vi "Check Generation Status.vi"(0 "fpga interface in":refnum<k20>, 11 "error in (no error)":errorcluster) -> (4 "fpga interface out":refnum<k20>, 6 "generation done":bool, 8 "generation state":T1(ring), 15 "error out":errorcluster)   [LabVIEW 2023, in "GettingStarted_Gen_148X_Host.lvlib"]
uses:
  GettingStarted_Gen_148X_Host.lvlib
  <instrlib>/FlexRIO/CSI-2/v2/FPGA/Types/Generation Engine State.ctl
  <instrlib>/FlexRIO/CSI-2/v2/FPGA/NI CSI-2 API FPGA v2.lvlib
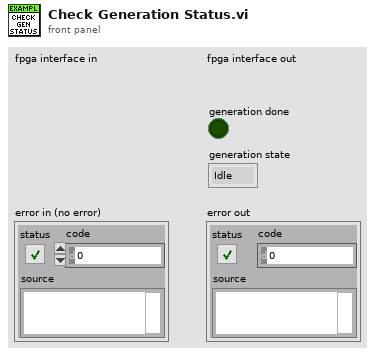
[diagram p1: front panel]
types:
  T1 = enum8{"Idle", "Ready For Start Trigger", "Generate Packets", "Done", "Error"}
  T2 = typedef "NI CSI-2 API FPGA v2.lvlib/Generation Engine State.ctl" = enum8{"Idle", "Ready For Start Trigger", "Generate Packets", "Done", "Error"}
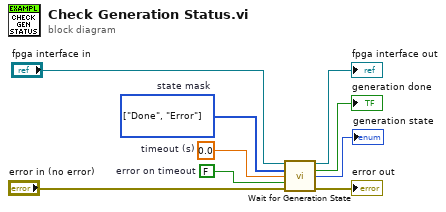
[diagram p0: block diagram]
diagram:
  w4 = FALSE  # error on timeout
  w5 = 0.0  # timeout (s)
  w6 = T2[] [enum."Done", enum."Error"] items=["Idle", "Ready For Start Trigger", "Generate Packets", "Done", "Error"]  # state mask
  n1 = call "Wait for Generation State.vi"("fpga interface in"="fpga interface in", "state mask"=w6, "timeout (s)"=w5, "error on timeout"=w4, "error in (no error)"="error in (no error)") -> ("fpga interface out"=→"fpga interface out":refnum<k20>, "state matches"=→"generation done":bool, "state"=→"generation state":T1, "error out"=→"error out":errorcluster)  [unwired: 7 in]
